vi "Build Rotation Set.vi"(7 "Rotate(Yaw) CCW 1 CW -1":dbl, 11 "Frame Set":T1 {"Back Right"."Angle" scale format="%.3f"; "Back Right"."Velocity" scale=-1.0..1.0 scale format="%.1f"; "Back Left"."Angle" scale format="%.3f"; "Back Left"."Velocity" scale=-1.0..1.0 scale format="%.1f"; "Front Left"."Angle" scale format="%.3f"; "Front Left"."Velocity" scale=-1.0..1.0 scale format="%.1f"; "Front Right"."Angle" scale format="%.3f"; "Front Right"."Velocity" scale=-1.0..1.0 scale format="%.1f"}) -> (3 "Rotation Set Out":T1 {"Back Right"."Angle" scale format="%.3f"; "Back Right"."Velocity" scale=-1.0..1.0 scale format="%.1f"; "Back Left"."Angle" scale format="%.3f"; "Back Left"."Velocity" scale=-1.0..1.0 scale format="%.1f"; "Front Left"."Angle" scale format="%.3f"; "Front Left"."Velocity" scale=-1.0..1.0 scale format="%.1f"; "Front Right"."Angle" scale format="%.3f"; "Front Right"."Velocity" scale=-1.0..1.0 scale format="%.1f"})   [LabVIEW 2023, in "SwerveDrive_ACT_ts.lvlib"]
uses:
  SwerveDrive_ACT_ts.lvlib
  Shared Code/TypeDefs/Cluster_Swerve 4 Steer and Velocity.ctl
  Shared Code/TypeDefs/Cluster_Module Velocity-Direction-Rotations.ctl
  Shared Code/TypeDefs/Level_Velocity plus-minus 1.ctl
  Shared Code/TypeDefs/Dial_Compase heading unit circle CCW positive.ctl
panel:
  # "\"Front\" of Robot"
  # "Index 1"
  # "Index 0"
  # "Index 3"
  # "Index 2"
  # "Right Hand Rule"
  # "X"
  # "+CCW"
  # "Y"
  # "(0,0)"
  # "\"Front\" of Robot"
  # "Index 1"
  # "Index 0"
  # "Index 3"
  # "Index 2"
  # "Right Hand Rule"
  # "X"
  # "+CCW"
  # "Y"
  # "(0,0)"
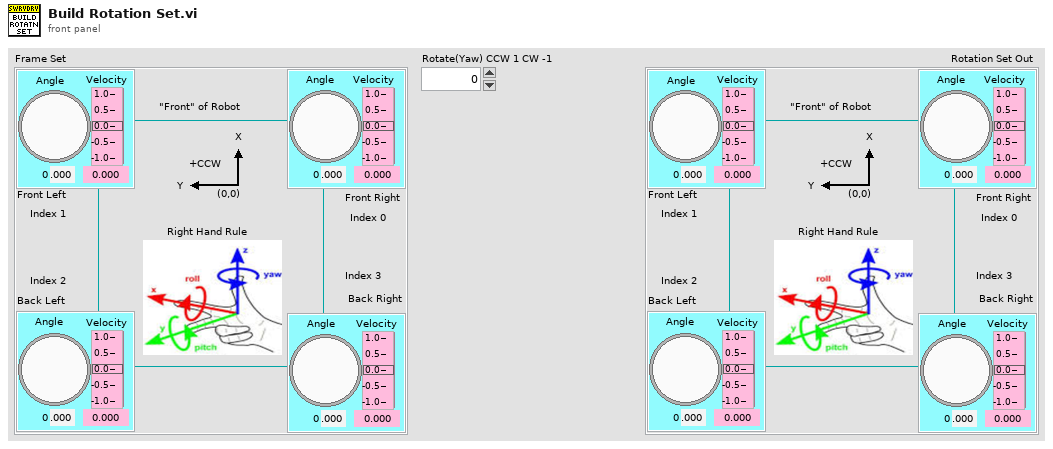
[diagram p1: front panel]
types:
  T1 = typedef "Cluster_Swerve 4 Steer and Velocity.ctl" = cluster{"Front Right":T2, "Front Left":T2, "Back Left":T2, "Back Right":T2}
  T2 = typedef "Cluster_Module Velocity-Direction-Rotations.ctl" = cluster{"Velocity":T3, "Angle":T4, "Rotations Count":dbl}
  T3 = typedef "Level_Velocity plus-minus 1.ctl" = dbl
  T4 = typedef "Dial_Compase heading unit circle CCW positive.ctl" = dbl
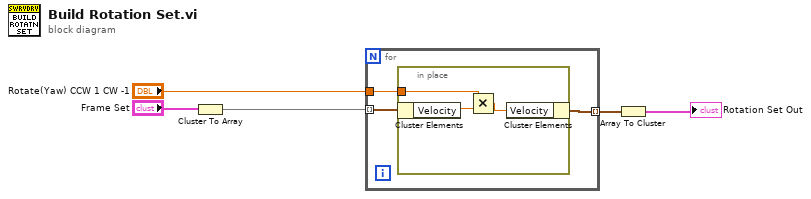
[diagram p0: block diagram]
diagram:
  n1 = Cluster To Array(cluster="Frame Set") -> (array=w4:T2[])
  n2 = for {
    tunnel: w4 -> [w8] mode=indexing
    tunnel: "Rotate(Yaw) CCW 1 CW -1" -> [w7]
    tunnel: [w6] -> w3 mode=indexing
    n3 = in-place {
      in-place-border: w7 -> [w9]
      n4 = in-place-cluster #1(w8) -> ("Velocity"=w11:T3)
      n5 = Multiply(x=w9, y=w11) -> (x*y=w10:T3)
      n6 = in-place-cluster #1("Velocity"=w10) -> (w6:T2)
    }
  }
  n7 = Array To Cluster(array=w3) -> (cluster=→"Rotation Set Out":cluster{"[0]":T2, "[1]":T2, "[2]":T2, "[3]":T2})
